vi "Get Cell Reference.vi"(8 "error in (no error)":errorcluster, 9 "y":i32, 10 "x":i32, 11 "map reference in":refnum<data-value>) -> (0 "error out":errorcluster, 1 "found?":bool, 2 "cell reference":refnum<data-value>, 3 "map reference out":refnum<data-value>)   [LabVIEW 2017, in "NI_Robotics_OccupancyGridWorldMap.lvclass"]
doc: "Returns a reference to the cell in the occupancy grid map at the position you specify."
uses:
  <vilib>/robotics/Navigation/shared/WorldMap/OccupancyGridWorldMap/NI_Robotics_OccupancyGridWorldMap.lvclass
  <vilib>/robotics/Navigation/shared/MapNode/OccupancyGridNode/NI_Robotics_OccupancyGridMapNode.lvclass
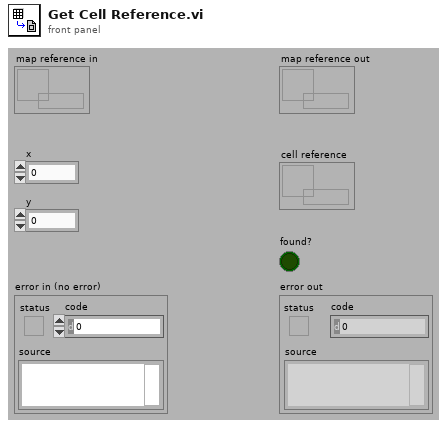
[diagram p1: front panel]
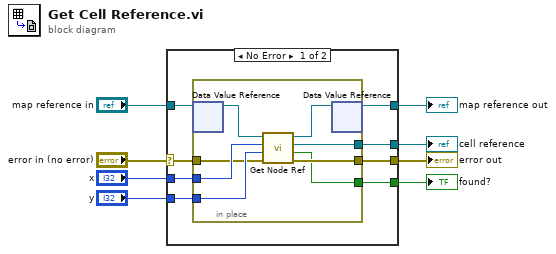
[diagram p0: block diagram]
diagram:
  n1 = case shown="No Error" "error in (no error)" {
    selector: "error in (no error)" -> [w13 w26]
    tunnel: [w12 w26] -> w7
    tunnel: "map reference in" -> [w16 w25]
    tunnel: "x" -> [w15 _]
    tunnel: "y" -> [w14 _]
    tunnel: [w11 _] -> w3
    tunnel: [w10 _] -> w2
    tunnel: [w9 w25] -> w1
    frame No Error {
      n2 = in-place {
        in-place-border: w15 -> [w23]
        in-place-border: w14 -> [w22]
        in-place-border: w13 -> [w21]
        in-place-border: [w19] -> w12
        in-place-border: [w18] -> w11
        in-place-border: [w17] -> w10
        n3 = in-place-dvr #1(w16) -> (w24:refnum<class "NI_Robotics_OccupancyGridWorldMap.lvclass">)  [unwired: 1 out]
        n4 = call <vilib>:"Get Node Ref.vi"("error in (no error)"=w21, "y"=w22, "x"=w23, "OccupancyGridWorldMap in"=w24) -> ("error out"=w19:errorcluster, "Found"=w17:bool, "element"=w18:refnum<data-value>, "OccupancyGridWorldMap out"=w20:refnum<class "NI_Robotics_OccupancyGridWorldMap.lvclass">)  [unwired: 4 in]
        n5 = in-place-dvr #1(w20) -> (w9:refnum<data-value>)  [unwired: 1 out]
      }
    }
    frame Error {
    }
  }
  "map reference out" <- w1
  "error out" <- w7
  "cell reference" <- w3
  "found?" <- w2
